vi "Dequeue Message.vi"(8 "error in (no error)":errorcluster, 11 "Queue In":T1) -> (0 "error out":errorcluster, 1 "Message Data":variant, 2 "Message":string, 3 "Queue Out":T1, 5 "timed out?":bool)   [LabVIEW 2023, in "VeriStand Console.lvlib"]
uses:
  VeriStand Console.lvlib
  Message Queue.ctl
  Message.ctl
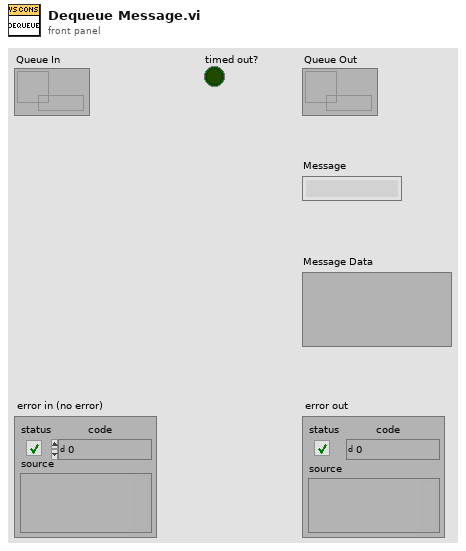
[diagram p1: front panel]
types:
  T1 = typedef "VeriStand Console.lvlib/Message Queue.ctl" = refnum<queue>
  T2 = typedef "VeriStand Console.lvlib/Message.ctl" = cluster{"Message":string, "Message Data":variant}
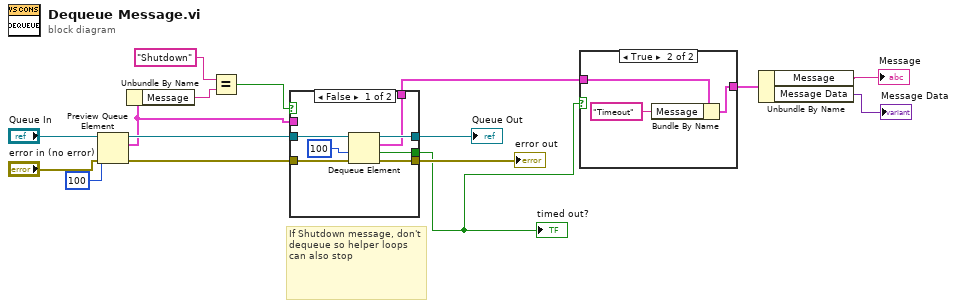
[diagram p0: block diagram]
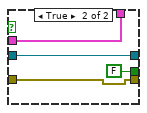
[diagram p2: hidden frame]
diagram:
  # "If Shutdown message, don't dequeue so helper loops can also stop"
  n1 = Preview Queue Element(queue="Queue In", timeout in ms (-1)=100, error in (no error)="error in (no error)") -> (queue out=w8:T1, element=w3:T2, error out=w2:errorcluster)  [unwired: 1 out]
  n2 = Unbundle By Name(w3) -> ("Message"=w6:string)
  n3 = Equal?(x="Shutdown" ("Message"), y=w6) -> (x = y?=w4:bool)
  n4 = case shown="False" w4 {
    tunnel: [w23 w26] -> w16
    tunnel: [w22 w24] -> w15
    tunnel: [w20 w27] -> w12
    tunnel: [w19 FALSE ("timed out?")] -> w11
    tunnel: w8 -> [w18 w26]
    tunnel: w3 -> [_ w27]
    tunnel: w2 -> [w17 w24]
    frame False {
      n5 = Dequeue Element(queue=w18, timeout in ms (-1)=100, error in (no error)=w17) -> (queue out=w23:T1, element=w20:T2, timed out?=w19:bool, error out=w22:errorcluster)
    }
    frame True {
    }
  }
  "error out" <- w15
  "Queue Out" <- w16
  "timed out?" <- w11
  n6 = case shown="True" w11 {
    tunnel: w12 -> [w28 w31]
    tunnel: [w28 w30] -> w10
    frame False {
    }
    frame True {
      n7 = Bundle By Name(cluster=w31, "Message"="Timeout") -> (w30:T2)
    }
  }
  n8 = Unbundle By Name(w10) -> ("Message"=→"Message":string, "Message Data"=→"Message Data":variant)
